vi "Get Result.vi"(8 "error in (no error)":errorcluster, 11 "Red Pitaya Lock-in Driver in":refnum<class "Red Pitaya Lock-in Driver.lvclass">) -> (0 "error out":errorcluster, 2 "Result":refnum<class "Acquired Result.lvclass">, 3 "Red Pitaya Lock-in Driver out":refnum<class "Red Pitaya Lock-in Driver.lvclass">)   [LabVIEW 2016, in "Red Pitaya Lock-in Driver.lvclass"]
uses:
  Red Pitaya Lock-in Driver.lvclass
  C:/github/NHMFL_Core/Libraries/Instruments/Instrument Driver/Lock-in Driver/Lock-in Driver.lvclass
  C:/github/NHMFL_Core/Libraries/Instruments/Instrument Driver/Instrument Driver.lvclass
  LabActor/Results/Acquired Result/Acquired Result.lvclass
  Red Pitaya Lock-in Driver.lvclass/Red Pitaya Lock-in Driver.ctl
  Instruments/Instrument Driver/Instrument Driver.lvclass/Instrument Driver.ctl
  <vilib>/express/express signal manip/GetorSetDDTAttributes/Shared VIs/TimeType.ctl
  LabActor/Results/Acquired Result/Acquired Result.lvclass/Acquired Result.ctl
  Read RP Instrument.vi
  Instruments/Instrument Driver/Read Recorder name.vi
  Instruments/Instrument Driver/Read Group name.vi
  Write RP Instrument.vi
  LabActor/Results/Acquired Result/Write Channels.vi
  LabActor/Results/Acquired Result/Write Group.vi
  Instruments/Instrument Driver/Lock-in Driver/Read Lock-in configuration.vi
  <vilib>/express/express signal manip/GetorSetDDTAttributes/Shared VIs/TimeMode Enum to Boolean.vi
  <vilib>/express/express shared/transition.llb/Dynamic To Waveform Array.vi
  <vilib>/express/express signal manip/GetorSetDDTAttributes/Set DDT Attributes/SetT0.vi
  <vilib>/express/express shared/transition.llb/Waveform Array To Dynamic.vi
  RP Instrument/RP Instrument.lvclass
  <vilib>/express/express signal manip/GetorSetDDTAttributes/Set DDT Attributes/Set DDT Properties.xnode
  <vilib>/express/express signal manip/GetorSetDDTAttributes/Shared VIs/GetSetShared.lvlib
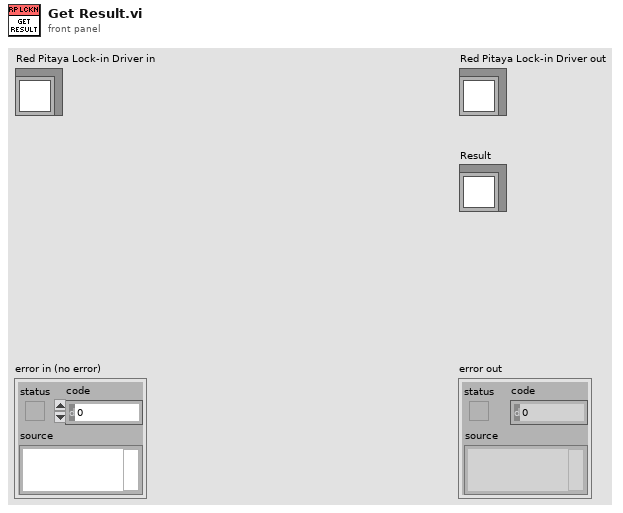
[diagram p1: front panel]
types:
  T1 = typedef "Lock-in Configuration.ctl" = cluster{"Frequency":dbl, "Time constant":dbl, "Synchronous":bool, "Channels":i32[]}
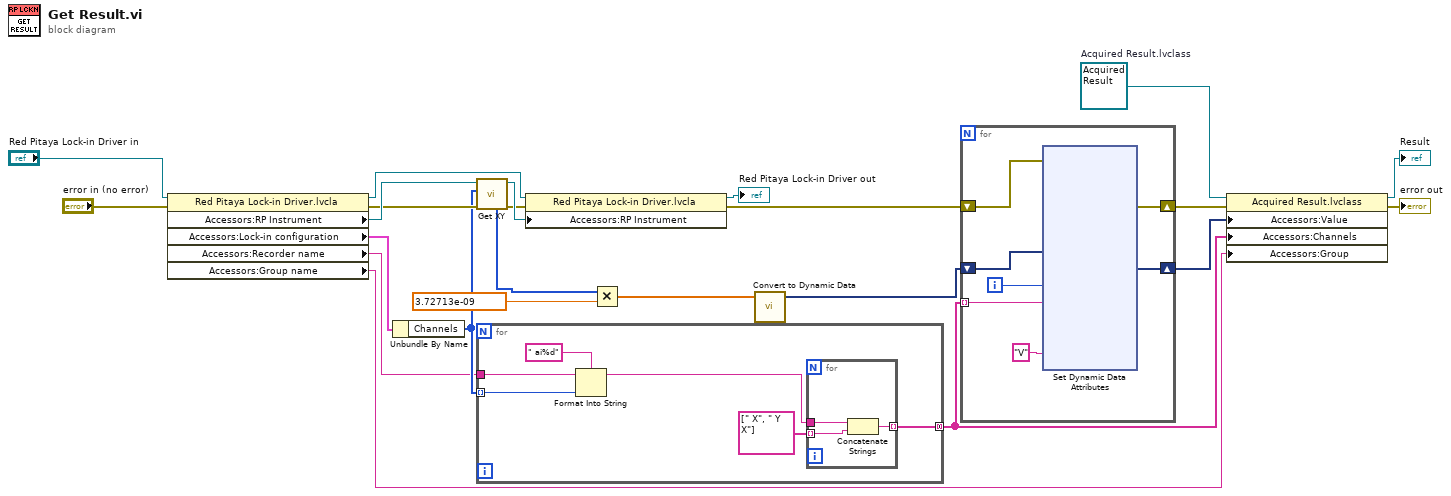
[diagram p0: block diagram]
diagram:
  w13 = refnum<class "Acquired Result.lvclass"> refnum  # Acquired Result.lvclass
  n1 = property class="Red Pitaya Lock-in Driver.lvcla"(reference="Red Pitaya Lock-in Driver in", error in="error in (no error)") -> (reference out=w20:refnum<class "Red Pitaya Lock-in Driver.lvclass">, error out=w18:errorcluster, "Accessors:RP Instrument"=w22:refnum<class "RP Instrument.lvclass">, "Accessors:Lock-in configuration"=w5:T1, "Accessors:Recorder name"=w2:string, "Accessors:Group name"=w6:string)
  n2 = Unbundle By Name(w5) -> ("Channels"=w3:i32[])
  n3 = call-dynamic "Get XY.vi"("error in (no error)"=w18, "Channels"=w3, "RP Instrument in"=w22) -> ("error out"=w10:errorcluster, "RP Instrument out"=w21:refnum<class "RP Instrument.lvclass">, "Signal"=w4:i32[])  [unwired: 6 in]
  n4 = for {
    tunnel: w3 -> [w24] mode=indexing
    tunnel: w2 -> [w28]
    tunnel: [w25] -> w1 mode=concatenating
    n5 = Format Into String(format string=" ai%d", initial string=w28, w24) -> (resulting string=w26:string)  [unwired: 1 in, 1 out]
    n6 = for {
      tunnel: string[] [" X", " Y X"] -> [w32] mode=indexing
      tunnel: w26 -> [w31]
      tunnel: [w30] -> w25 mode=indexing
      n7 = Concatenate Strings(w31, w32) -> (w30:string)
    }
  }
  n8 = property class="Red Pitaya Lock-in Driver.lvcla"(reference=w20, error in=w10, "Accessors:RP Instrument"=w21) -> (reference out=→"Red Pitaya Lock-in Driver out":refnum<class "Red Pitaya Lock-in Driver.lvclass">, error out=w11:errorcluster)
  n9 = Multiply(x=w4, y=3.72713e-09) -> (x*y=w16:dbl[])
  n10 = call "Convert to Dynamic Data"("Array"=w16) -> ("Dynamic Data Type"=w15:dynamicdata)  [unwired: 3 in]
  n11 = for {
    tunnel: w1 -> [w37] mode=indexing
    shift-right: [w35] -> w14
    shift-left: w15 -> [w38]
    shift-right: [w34] -> w12
    shift-left: w11 -> [w33]
    i -> [w39]
    n12 = xnode "Set Dynamic Data Attributes"("Signals In"=w38, "Signal Index"=w39, "Signal Name"=w37, "Unit"="V", "error in"=w33) -> ("Signals Out"=w35:dynamicdata, "error out"=w34:errorcluster)  [unwired: 2 in]
  }
  n13 = property class="Acquired Result.lvclass"(reference=w13, error in=w12, "Accessors:Value"=w14, "Accessors:Channels"=w1, "Accessors:Group"=w6) -> (reference out=→"Result":refnum<class "Acquired Result.lvclass">, error out=→"error out":errorcluster)
